vi "Handle Plugin Errors.vi"(8 "error in (no error)":errorcluster, 11 "Invalid Plugin Array":T1[](array[typedef])) -> (0 "error out":errorcluster)   [LabVIEW 2020, in "RxnRover.lvlib" / "Plugin Manager.lvlib"]
doc: "Handles RxnRover plugin errors by displayig a dialog message including list of the invalid plugin names in the RxnRover menu and logs the details of any errors in a .txt file (pluginerrors.txt)\n\nCreated:\nRxnRover\nMay 26, 2025"
uses:
  Plugin Manager.lvlib
  Plugin Details.ctl
  Plugin Servers/Controller/Controller Type.ctl
  Plugin Types.ctl
  Config Error.ctl
  File IO/File IO.lvlib
  File IO/Project Locations/Project Locations.lvlib
  Plugin Servers/Controller/Generic Plugin.lvclass
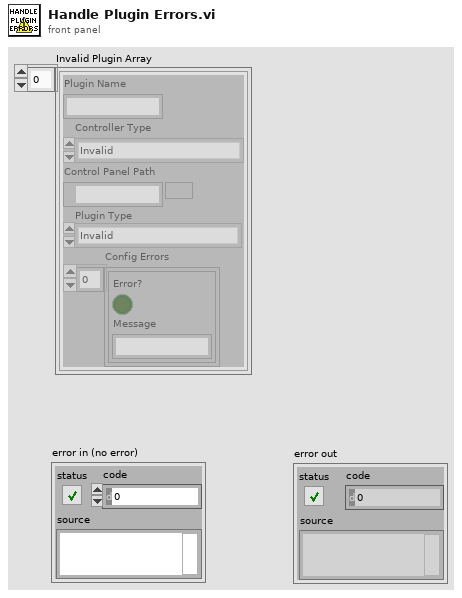
[diagram p1: front panel]
types:
  T1 = typedef "RxnRover.lvlib/Plugin Manager.lvlib/Plugin Details.ctl" = cluster{"Plugin Name":string, "Controller Type":T2, "Control Panel Path":path, "Plugin Type":T3, "Config Errors":T4[]}
  T2 = typedef "RxnRover.lvlib/Generic Plugin.lvclass/Controller Type.ctl" = enum16{"Invalid", "Temperature Controller", "Pump Controller", "Syringe Pump", "Generic Optimizer", "LC Parser", "Passive Hardware"}
  T3 = typedef "RxnRover.lvlib/Plugin Manager.lvlib/Plugin Types.ctl" = enum16{"Invalid", "Optimizer", "Analyzer", "Hardware"}
  T4 = typedef "RxnRover.lvlib/Plugin Manager.lvlib/Config Error.ctl" = cluster{"Error?":bool, "Message":string}
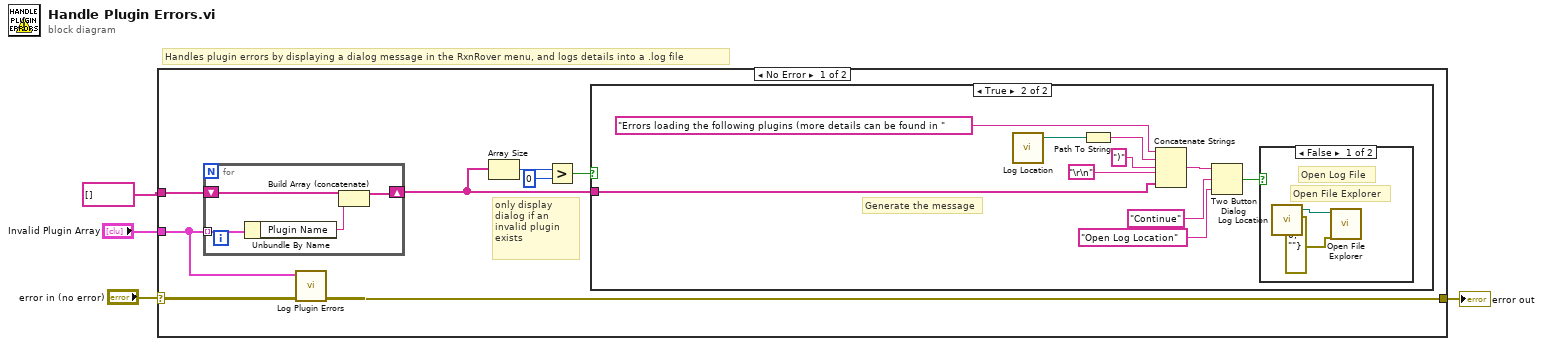
[diagram p0: block diagram]
diagram:
  # "Handles plugin errors by displaying a dialog message in the RxnRover menu, and logs details into a .log file"
  n1 = case shown="No Error" "error in (no error)" {
    selector: "error in (no error)" -> [w7 w29]
    tunnel: "Invalid Plugin Array" -> [w5 _]
    tunnel: string[] [] -> [w12 _]
    tunnel: [w6 w29] -> w1
    frame No Error {
      # "only display dialog if an invalid plugin exists"
      n2 = for {
        tunnel: w5 -> [w28] mode=indexing
        shift-right: [w27] -> w8
        shift-left: w12 -> [w26]
        n3 = Unbundle By Name(w28) -> ("Plugin Name"=w25:string)
        n4 = Build Array (concatenate)(w26, w25) -> (w27:string[])
      }
      n5 = call "Log Plugin Errors.vi"("error in (no error)"=w7, "Full Plugin Array"=w5) -> ("error out"=w6:errorcluster)  [unwired: 9 in]
      n6 = Array Size(array=w8) -> (size(s)=w11:i32)
      n7 = Greater?(x=w11, y=0) -> (0:w9:bool)
      n8 = case shown="True" w9 {
        tunnel: w8 -> [_ w21]
        frame False {
        }
        frame True {
          # "Generate the message"
          n9 = call "Log Location.vi"() -> ("Log Location"=w16:path)  [unwired: 2 in]
          n10 = Path To String(path=w16) -> (string=w15:string)
          n11 = Concatenate Strings("Errors loading the following plugins (more details can be found in " ("string"), w15, ")" ("string"), "\r\n", w21) -> (w22:string)
          n12 = Two Button Dialog(message=w22, 1:"Open Log Location" ("F button name (\"Cancel\")"), 2:"Continue" ("T button name (\"OK\")")) -> (T button?=w18:bool)
          n13 = case shown="False" w18 {
            frame False {
              # "Open Log File"
              # "Open File Explorer"
              n14 = call "Log Location.vi"() -> ("Log Location"=w23:path)  [unwired: 2 in]
              n15 = call "Open File Explorer.vi"("error in (no error)"=errorcluster {"status"=FALSE, "code"=0, "source"=""}, "Full Path"=w23) -> ()  [unwired: 9 in, 1 out]
            }
            frame True {
              # "Continue"
            }
          }
        }
      }
    }
    frame Error {
    }
  }
  "error out" <- w1
